vi "Prepare calendar.vi"(0 "Month ctrl":i32, 5 "Year ctrl":i32, 7 "Find day of the month index":i32) -> (4 "Array":string[][](array[string]), 6 "date time rec":T2, 8 "Day of the month index":T1)   [LabVIEW 2011, in "Calendar XControl.xctl"]
uses:
  Calendar XControl.xctl
  <vilib>/Utility/miscctls.llb/LVDateTimeRec.ctl
  <vilib>/Utility/miscctls.llb/LVRowAndColumnTypeDef.ctl
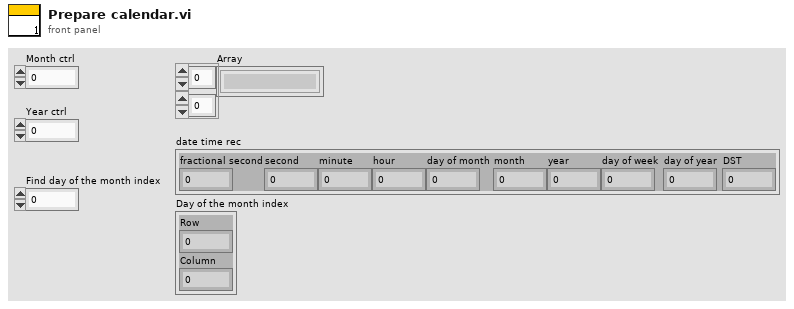
[diagram p1: front panel]
types:
  T1 = typedef "LVRowAndColumnTypeDef.ctl" = cluster{"Row":i32, "Column":i32}
  T2 = typedef "LVDateTimeRec.ctl" = cluster{"fractional second":dbl, "second":i32, "minute":i32, "hour":i32, "day of month":i32, "month":i32, "year":i32, "day of week":i32, "day of year":i32, "DST":i32}
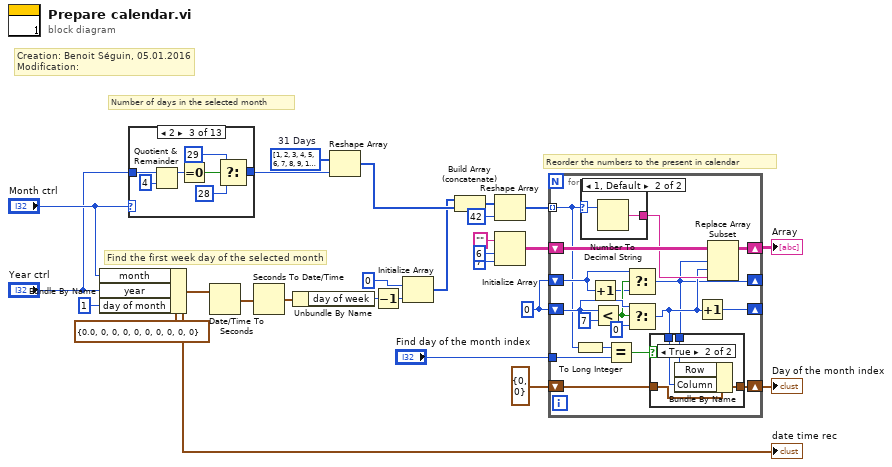
[diagram p0: block diagram]
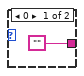
[diagram p3: hidden frame]
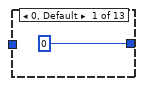
[diagram p4: hidden frame]
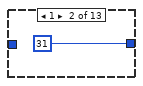
[diagram p5: hidden frame]
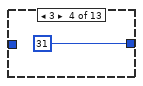
[diagram p6: hidden frame]
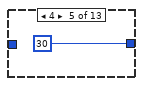
[diagram p7: hidden frame]
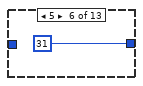
[diagram p8: hidden frame]
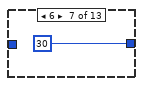
[diagram p9: hidden frame]
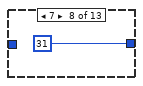
[diagram p10: hidden frame]
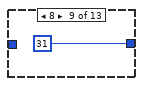
[diagram p11: hidden frame]
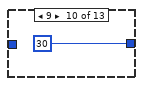
[diagram p12: hidden frame]
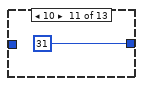
[diagram p13: hidden frame]
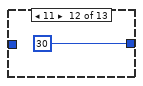
[diagram p14: hidden frame]
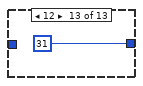
[diagram p15: hidden frame]
diagram:
  w11 = 0
  w20 = u8[] [1, 2, 3, 4, 5, 6, 7, 8, 9, 10, 11, 12, 13, 14, 15, 16, 17, 18, 19, 20, 21, 22, 23, 24, 25, 26, 27, 28, 29, 30, 31]  # 31 Days
  # "Creation: Benoit Séguin, 05.01.2016\nModification:"
  # "Reorder the numbers to the present in calendar"
  # "Number of days in the selected month"
  # "Find the first week day of the selected month"
  n1 = Bundle By Name(cluster=T2 {"fractional second"=0.0, "second"=0, "minute"=0, "hour"=0, "day of month"=0, "month"=0, "year"=0, "day of week"=0, "day of year"=0, "DST"=0} ("date time rec"), "month"="Month ctrl", "year"="Year ctrl", "day of month"=1) -> (w4:T2)
  "date time rec" <- w4
  n2 = case shown="2" "Month ctrl" {
    tunnel: [0 ("t") 31 w29 31 30 31 30 31 31 30 31 30 31] -> w19
    tunnel: "Year ctrl" -> [_ _ w33 _ _ _ _ _ _ _ _ _ _]
    frame 0, Default {
    }
    frame 1 {
    }
    frame 2 {
      n3 = Quotient & Remainder(x=w33, y=4) -> (x-y*floor(x/y)=w34:i32)  [unwired: 1 out]
      n4 = Equal To 0?(x=w34) -> (x = 0?=w32:bool)
      n5 = Select(t=29, s=w32, f=28) -> (s? t:f=w29:i32)
    }
    frame 3 {
    }
    frame 4 {
    }
    frame 5 {
    }
    frame 6 {
    }
    frame 7 {
    }
    frame 8 {
    }
    frame 9 {
    }
    frame 10 {
    }
    frame 11 {
    }
    frame 12 {
    }
  }
  n6 = Date/Time To Seconds(2:w4) -> (0:w24:timestamp)  [unwired: 1 in]
  n7 = Seconds To Date/Time(time stamp (now)=w24) -> (date time rec=w25:T2)  [unwired: 1 in]
  n8 = Unbundle By Name(w25) -> ("day of week"=w18:i32)
  n9 = Reshape Array(w20, w19) -> (w16:u8[])
  n10 = Decrement(x=w18) -> (x-1=w5:i32)
  n11 = Initialize Array(u8 0, w5) -> (w15:u8[])
  n12 = Build Array (concatenate)(w15, w16) -> (w14:u8[])
  n13 = Reshape Array(w14, 42 ("dimension size")) -> (w12:u8[])
  n14 = Initialize Array("", 6 ("dimension size"), 7 ("dimension size")) -> (w7:string[][])
  n15 = for {
    tunnel: w12 -> [w53] mode=indexing
    shift-right: [w60] -> _
    shift-left: w11 -> [w62]
    shift-right: [w47] -> _
    shift-left: w11 -> [w57]
    shift-right: [w56] -> w6
    shift-left: w7 -> [w55]
    tunnel: "Find day of the month index" -> [w52]
    shift-right: [w49] -> w1
    shift-left: T1 {"Row"=0, "Column"=0} ("CellPosition") -> [w50]
    n16 = To Long Integer(number=w53) -> (32bit integer=w46:i32)
    n17 = case shown="1, Default" w53 {
      selector: w53 -> [_ w71]
      tunnel: ["" w70] -> w54
      frame 0 {
      }
      frame 1, Default {
        n18 = Number To Decimal String(number=w71) -> (decimal integer string=w70:string)  [unwired: 1 in]
      }
    }
    n19 = Increment(x=w57) -> (x+1=w58:i32)
    n20 = Less?(x=w62, y=7) -> (x < y?=w59:bool)
    n21 = Equal?(x=w46, y=w52) -> (x = y?=w51:bool)
    n22 = Select(t=w57, s=w59, f=w58) -> (s? t:f=w47:i32)
    n23 = Select(t=w62, s=w59, f=0) -> (s? t:f=w48:i32)
    n24 = case shown="True" w51 {
      tunnel: w50 -> [w64 w67]
      tunnel: [w64 w68] -> w49
      tunnel: w48 -> [_ w65]
      tunnel: w47 -> [_ w66]
      frame False {
      }
      frame True {
        n25 = Bundle By Name(cluster=w67, "Row"=w66, "Column"=w65) -> (w68:T1)
      }
    }
    n26 = Increment(x=w48) -> (x+1=w60:i32)
    n27 = Replace Array Subset(array=w55, new element=w54, index (row)=w47, index (col)=w48) -> (w56:string[][])
  }
  "Array" <- w6
  "Day of the month index" <- w1
